vi "Get Output.vi"(8 "error in (no error)":errorcluster, 11 "Stanford Research PS350 in":refnum<class "Stanford Research PS350.lvclass">) -> (0 "error out":errorcluster, 2 "output":bool, 3 "Stanford Research PS350 out":refnum<class "Stanford Research PS350.lvclass">)   [LabVIEW 2011, in "Stanford Research PS350.lvclass"]
uses:
  Stanford Research PS350.lvclass
  Stanford Research PS350.lvclass/Stanford Research PS350.ctl
panel:
  out "read buffer":string
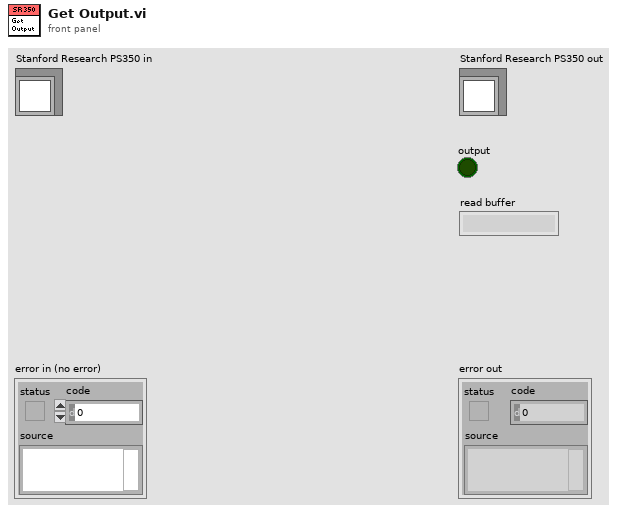
[diagram p1: front panel]
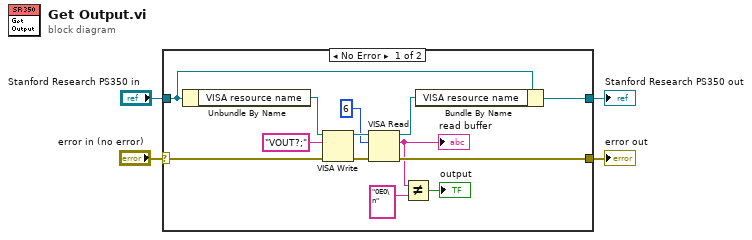
[diagram p0: block diagram]
diagram:
  n1 = case shown="No Error" "error in (no error)" {
    selector: "error in (no error)" -> [w15 w19]
    tunnel: [w9 w19] -> w3
    tunnel: [w8 w18] -> w1
    tunnel: "Stanford Research PS350 in" -> [w17 w18]
    frame No Error {
      n2 = Unbundle By Name(w17) -> ("VISA resource name"=w16:refnum<visa-resource-name>)
      n3 = VISA Write(VISA resource name=w16, write buffer="VOUT?;", error in (no error)=w15) -> (VISA resource name out=w13:refnum<visa-resource-name>, error out=w12:errorcluster)  [unwired: 1 out]
      n4 = VISA Read(VISA resource name=w13, byte count=u32 6, error in (no error)=w12) -> (VISA resource name out=w10:refnum<visa-resource-name>, read buffer=w6:string, error out=w9:errorcluster)  [unwired: 1 out]
      "read buffer" <- w6
      n5 = Not Equal?(x=w6, y="0E0\n" ("read buffer")) -> (x != y?=→"output":bool)
      n6 = Bundle By Name(cluster=w17, "VISA resource name"=w10) -> (w8:refnum<class "Stanford Research PS350.lvclass">)
    }
    frame Error {
    }
  }
  "error out" <- w3
  "Stanford Research PS350 out" <- w1
